vi "Send Sync.vi"(8 "error in (no error)":errorcluster, 11 "LINX-ADS1256 in":refnum<class "LINX-ADS1256.lvclass">) -> (0 "error out":errorcluster, 3 "LINX-ADS1256 out":refnum<class "LINX-ADS1256.lvclass">)   [LabVIEW 2020, in "LINX-ADS1256.lvclass"]
uses:
  LINX-ADS1256.lvclass
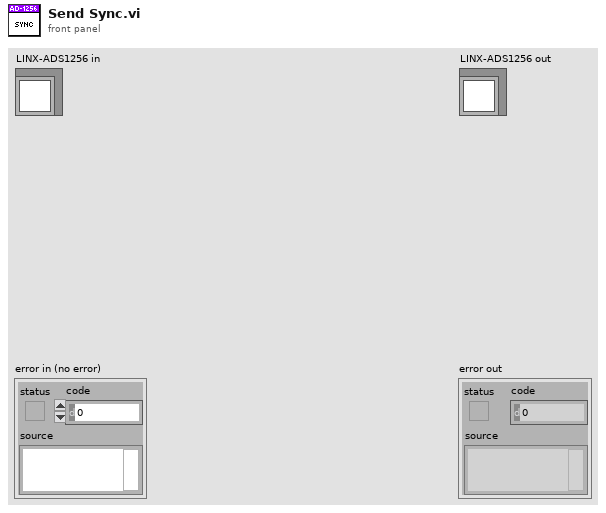
[diagram p1: front panel]
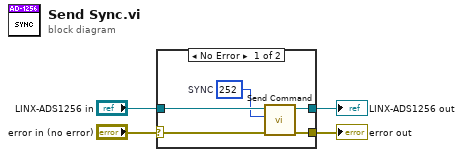
[diagram p0: block diagram]
diagram:
  n1 = case shown="No Error" "error in (no error)" {
    selector: "error in (no error)" -> [w7 w11]
    tunnel: [w6 w11] -> w3
    tunnel: [w8 w10] -> w1
    tunnel: "LINX-ADS1256 in" -> [w9 w10]
    frame No Error {
      w5 = u8 252  # SYNC
      n2 = call "Send Command.vi"("error in (no error)"=w7, "Register Address"=w5, "LINX-ADS1256 in"=w9) -> ("error out"=w6:errorcluster, "LINX-ADS1256 out"=w8:refnum<class "LINX-ADS1256.lvclass">)  [unwired: 7 in]
    }
    frame Error {
    }
  }
  "error out" <- w3
  "LINX-ADS1256 out" <- w1
